vi "string to char array.vi"(1 "Stripped text":string) -> (0 "Array":string[](array[string]))   [LabVIEW 2018]
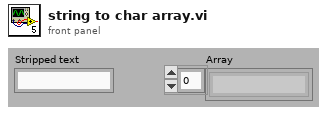
[diagram p1: front panel]
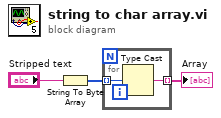
[diagram p0: block diagram]
diagram:
  n1 = String To Byte Array(string="Stripped text") -> (unsigned byte array=w1:u8[])
  n2 = for {
    tunnel: w1 -> [w5] mode=indexing
    tunnel: [w4] -> w2 mode=indexing
    n3 = Type Cast(x=w5) -> (*(type *) &x=w4:string)  [unwired: 1 in]
  }
  "Array" <- w2
